vi "AnalyzeHighRateVibrationData.vi"(8 "error in (no error)":errorcluster, 9 "data in":T7, 11 "Analysis Config":T1) -> (0 "error out":errorcluster, 1 "data out":T7, 3 "Analysis Config Out":T1)   [LabVIEW 2017, in "CmsAnalysisHighRate.lvlib"]
uses:
  <vilib>/addons/InsightCM/Devices/Shared/Cms/CmsAnalysisHighRate/CmsAnalysisHighRate.lvlib
  <vilib>/addons/InsightCM/Devices/Shared/Common/DataFlow/controls/Data.ctl
  <vilib>/addons/InsightCM/Utilities/DataAccessors/controls/wfmSGL_DVR.ctl
  <vilib>/addons/PointValueMap/controls/PointMap.ctl
  <vilib>/addons/InsightCM/Devices/Shared/Common/DataFlow/controls/Type.ctl
  <vilib>/addons/InsightCM/Devices/Shared/Cms/CmsAnalysis/controls/Config.ctl
  <vilib>/addons/InsightCM/Devices/Shared/Cms/CmsAnalysis/controls/Group.ctl
  <vilib>/addons/InsightCM/Utilities/Analysis/Shared/controls/Channel.ctl
  <vilib>/addons/InsightCM/Utilities/Analysis/Shared/controls/SpeedType.ctl
  <vilib>/addons/InsightCM/Utilities/Analysis/Shared/controls/Feature.ctl
  <vilib>/addons/InsightCM/Utilities/Analysis/Shared/controls/AmplitudeScale.ctl
  <vilib>/addons/InsightCM/Devices/Shared/Cms/CmsAnalysis/CmsAnalysis.lvlib
  <vilib>/addons/PointValueMap/PointValueMap.lvlib
  <vilib>/addons/InsightCM/Devices/Shared/Common/DataFlow/DataFlow.lvlib
  <vilib>/addons/InsightCM/Utilities/Analysis/Shared/AnalysisHelper.lvlib
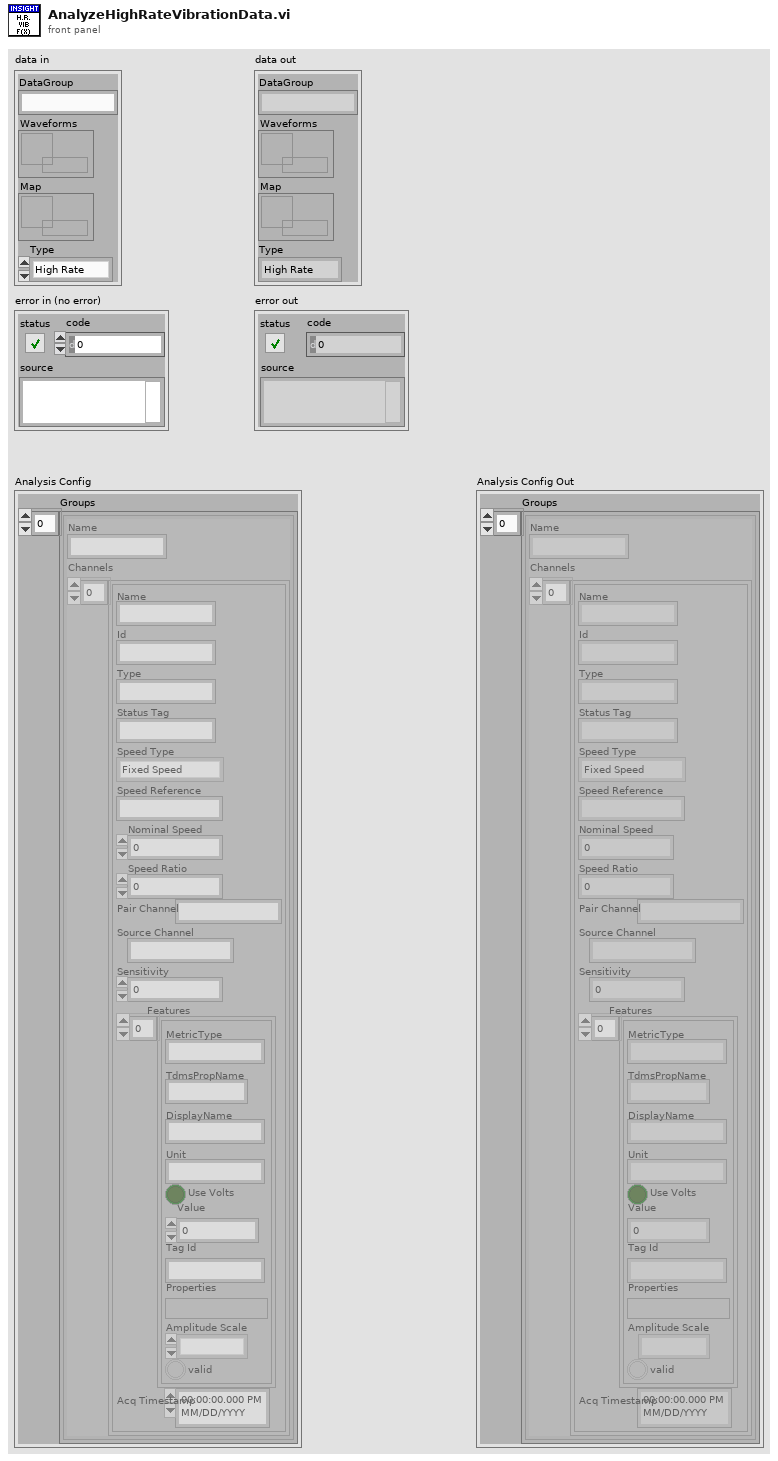
[diagram p1: front panel]
types:
  T1 = typedef "CmsAnalysis.lvlib/Config.ctl" = cluster{"Groups":T2[]}
  T2 = typedef "CmsAnalysis.lvlib/Group.ctl" = cluster{"Name":string, "Channels":T3[]}
  T3 = typedef "AnalysisHelper.lvlib/Channel.ctl" = cluster{"Name":string, "Id":string, "Type":string, "Status Tag":string, "Speed Type":T4, "Speed Reference":string, "Nominal Speed":dbl, "Speed Ratio":dbl, "Pair Channel":string, "Source Channel":string, "Sensitivity":dbl, "Features":T5[], "Acq Timestamp":timestamp}
  T4 = typedef "AnalysisHelper.lvlib/SpeedType.ctl" = enum16{"Fixed Speed", "Tachometer"}
  T5 = typedef "AnalysisHelper.lvlib/Feature.ctl" = cluster{"MetricType":string, "TdmsPropName":string, "DisplayName":string, "Unit":string, "Use Volts":bool, "Value":dbl, "Tag Id":string, "Properties":variant, "Amplitude Scale":T6, "valid":bool}
  T6 = typedef "AnalysisHelper.lvlib/AmplitudeScale.ctl" = enum16{"rms", "peak", "pk-pk"}
  T7 = typedef "DataFlow.lvlib/Data.ctl" = cluster{"DataGroup":string, "Waveforms":T8, "Map":T9, "Type":T10}
  T8 = typedef "wfmSGL_DVR.ctl" = refnum<data-value>
  T9 = typedef "PointValueMap.lvlib/PointMap.ctl" = refnum<data-value>
  T10 = typedef "DataFlow.lvlib/Type.ctl" = enum16{"High Rate", "Low Rate", "Burst Mode"}
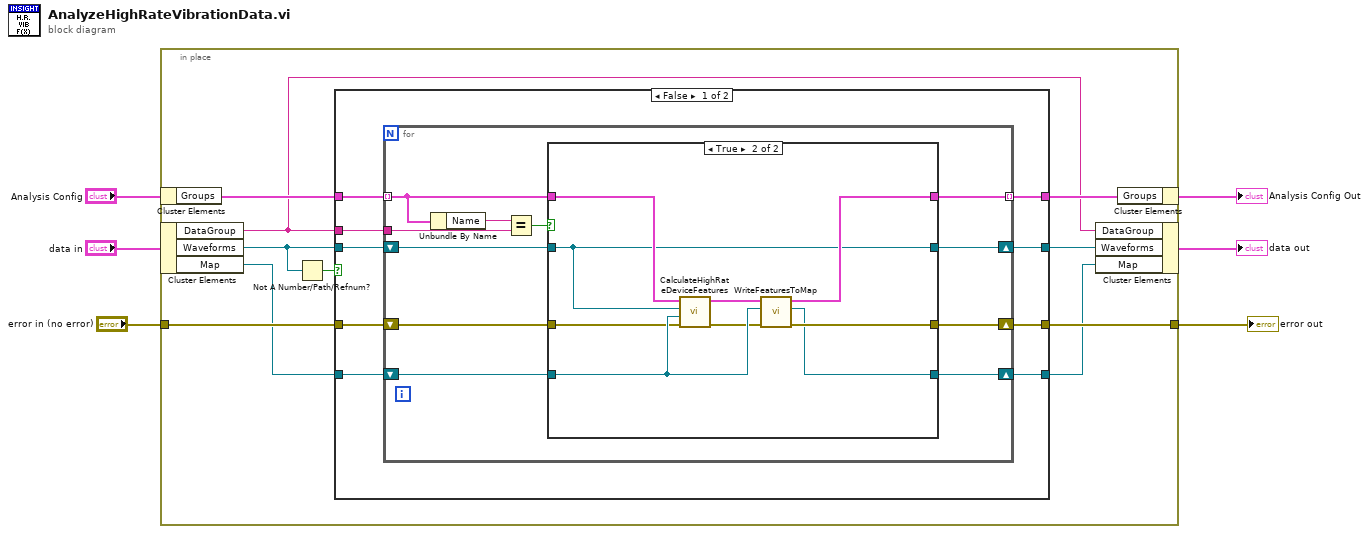
[diagram p0: block diagram]
diagram:
  n1 = in-place {
    in-place-border: [w16] -> w1
    in-place-border: "error in (no error)" -> [w13]
    n2 = in-place-cluster #1("Analysis Config") -> ("Groups"=w15:T2[])
    n3 = in-place-cluster #2("data in") -> ("DataGroup"=w10:string, "Waveforms"=w8:T8, "Map"=w12:T9)
    n4 = Not A Number/Path/Refnum?(number/path/refnum=w8) -> (NaN/Path/Refnum?=w7:bool)
    n5 = case shown="False" w7 {
      tunnel: [w25 w51] -> w16
      tunnel: w15 -> [w24 w53]
      tunnel: [w23 w53] -> w14
      tunnel: w13 -> [w22 w51]
      tunnel: w12 -> [w21 w50]
      tunnel: [w20 w52] -> w11
      tunnel: w10 -> [w19 _]
      tunnel: [w18 w50] -> w9
      tunnel: w8 -> [w17 w52]
      frame False {
        n6 = for {
          tunnel: w19 -> [w33]
          shift-right: [w36] -> w25
          shift-left: w22 -> [w32]
          tunnel: w24 -> [w29] mode=indexing
          tunnel: [w28] -> w23 mode=indexing
          shift-right: [w27] -> w20
          shift-left: w17 -> [w35]
          shift-right: [w26] -> w18
          shift-left: w21 -> [w34]
          n7 = Unbundle By Name(w29) -> ("Name"=w31:string)
          n8 = Equal?(x=w31, y=w33) -> (x = y?=w30:bool)
          n9 = case shown="True" w30 {
            tunnel: [w39 w49] -> w36
            tunnel: w35 -> [w38 w41]
            tunnel: w34 -> [w37 w48]
            tunnel: w32 -> [w39 w47]
            tunnel: w29 -> [w40 w46]
            tunnel: [w40 w45] -> w28
            tunnel: [w38 w41] -> w27
            tunnel: [w37 w44] -> w26
            frame False {
            }
            frame True {
              n10 = call <vilib>:"CalculateHighRateDeviceFeatures.vi"("error in (no error)"=w47, "Map"=w48, "Waveforms"=w41, "Group"=w46) -> ("error out"=w42:errorcluster, "Group out"=w43:T2)  [unwired: 6 in]
              n11 = call <vilib>:"WriteFeaturesToMap.vi"("error in (no error)"=w42, "Map in"=w48, "Group"=w43) -> ("error out"=w49:errorcluster, "Map out"=w44:T9, "Group out"=w45:T2)  [unwired: 6 in]
            }
          }
        }
      }
      frame True {
      }
    }
    n12 = in-place-cluster #2("DataGroup"=w10, "Waveforms"=w11, "Map"=w9) -> (→"data out":T7)
    n13 = in-place-cluster #1("Groups"=w14) -> (→"Analysis Config Out":T1)
  }
  "error out" <- w1
